vi "Logging Message Loop.vi"(8 "error in (no error)":errorcluster, 10 "Data Queue":refnum<queue>, 11 "Message Queues":T1) -> (0 "error out":errorcluster)   [LabVIEW 2020, in "Logging.lvlib"]
doc: "The message loop subVI to handle messages pertaining to logging data."
uses:
  Logging.lvlib
  MESSAGE_QUEUE/All Message Queues.ctl
  MESSAGE_QUEUE/Message Cluster.ctl
  SETTING/data_Queue.ctl
  Logging Configuration.ctl
  FITS/BigDataFits.ctl
  FITS/ClustBigFilFits.ctl
  FITS/DataTyp_Header.ctl
  MESSAGE_QUEUE/Message Queue.lvlib
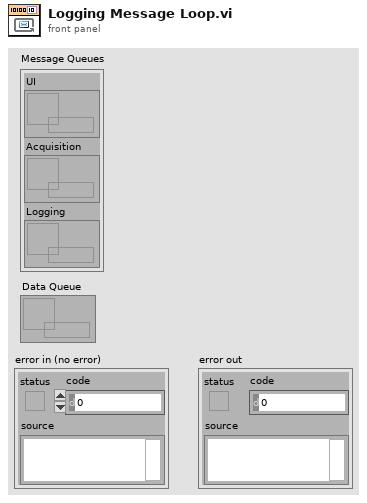
[diagram p1: front panel]
types:
  T1 = typedef "Message Queue.lvlib/All Message Queues.ctl" = cluster{"UI":refnum<queue>, "Acquisition":refnum<queue>, "Logging":refnum<queue>}
  T2 = typedef "Logging.lvlib/Logging Configuration.ctl" = cluster{"Log File Base Path":path, "NbrIma":i32}
  T3 = typedef "DataTyp_Header.ctl" = enum16{"U8 (unsigned integer 8bit)", "I16 (signed integer 16bit)", "U16 (unsigned integer 16 bit)", "I32 (signed integer 32bit)", "U32 (unsigned integer 32 bit)", "SGL (float 32bit)", "DBL(float 64bit)", "complex (2xfloat 64bit)"}
  T4 = typedef "ClustBigFilFits.ctl" = cluster{"file (use dialog)":path, "Type de données":T3, "Commentaire":string, "naxis1":i32, "naxis2":i32, "naxis3":i32, "Exptime":sgl}
  T5 = typedef "BigDataFits.ctl" = enum16{"Init", "WritHeader", "WritData", "Close"}
  T6 = typedef "data_Queue.ctl" = cluster{"tabIma":u16[][], "tabCdG":sgl[], "vectCom":sgl[]}
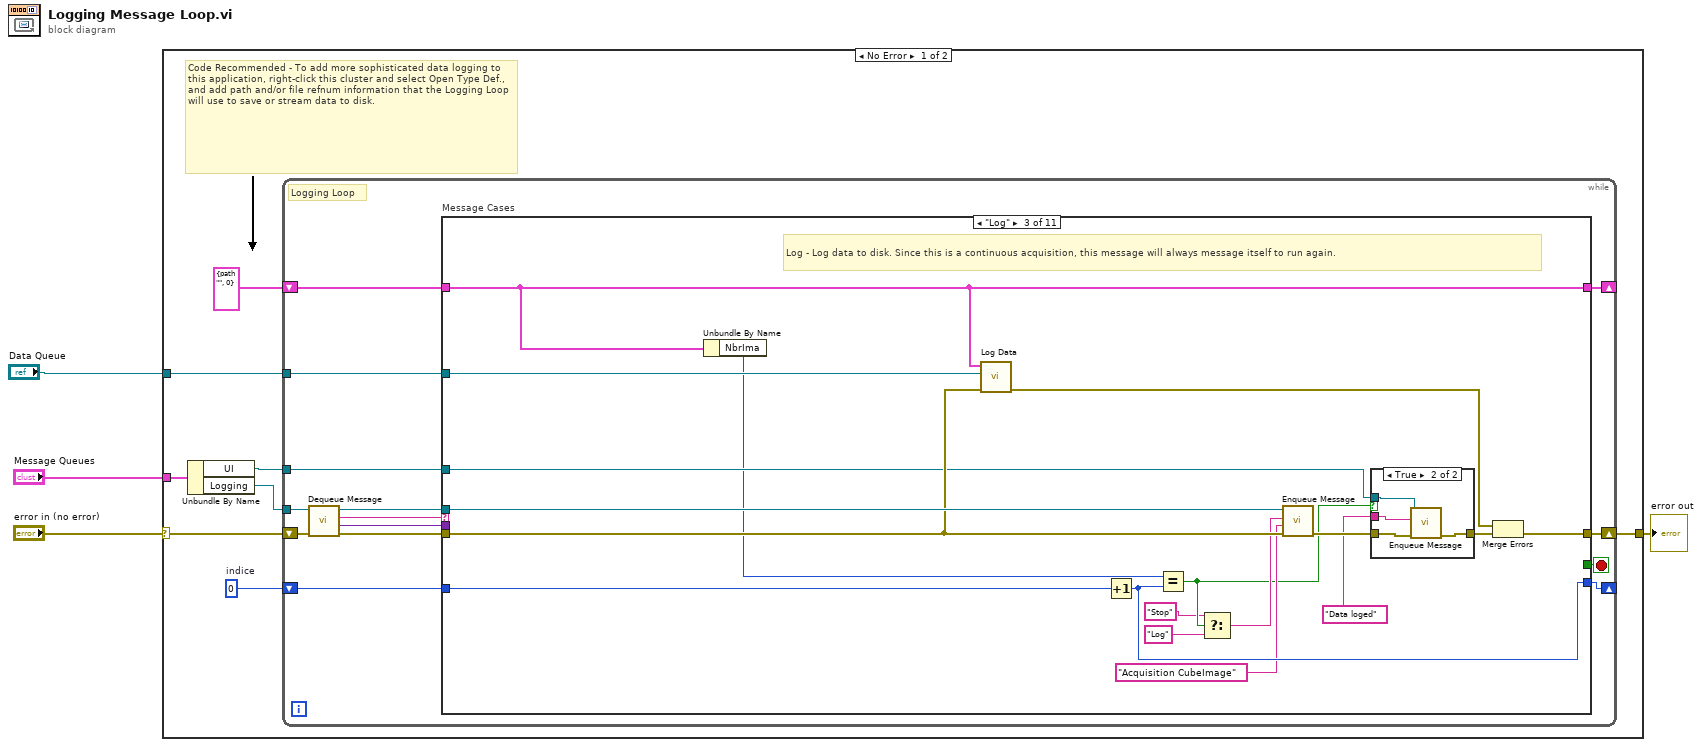
[diagram p0: block diagram]
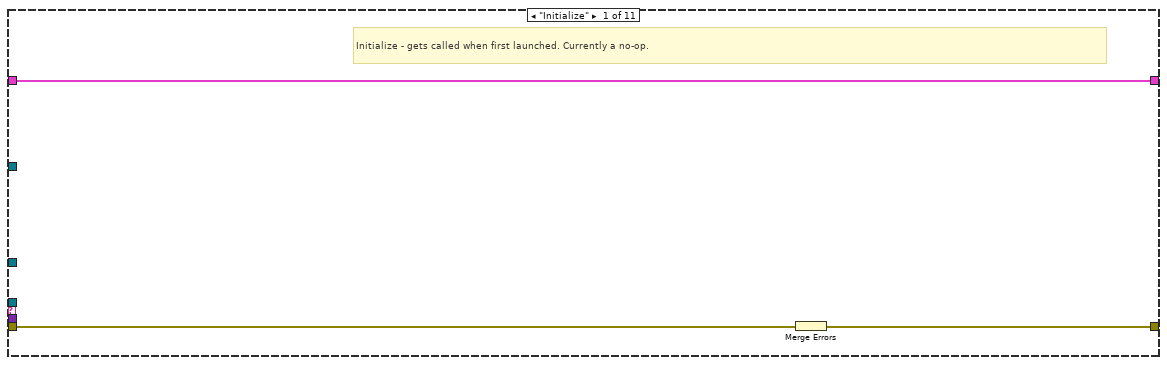
[diagram p2: hidden frame]
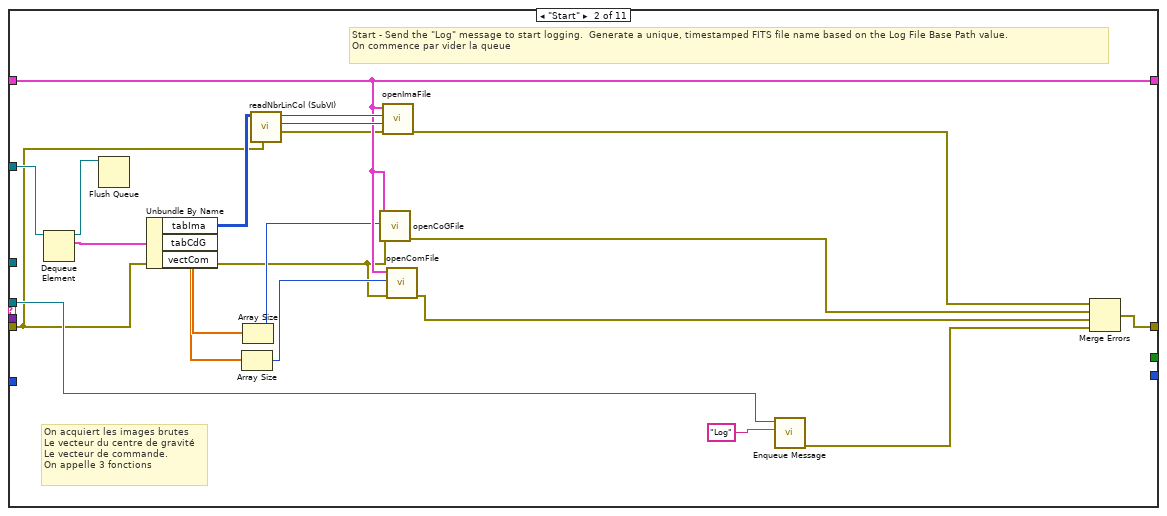
[diagram p3: hidden frame]
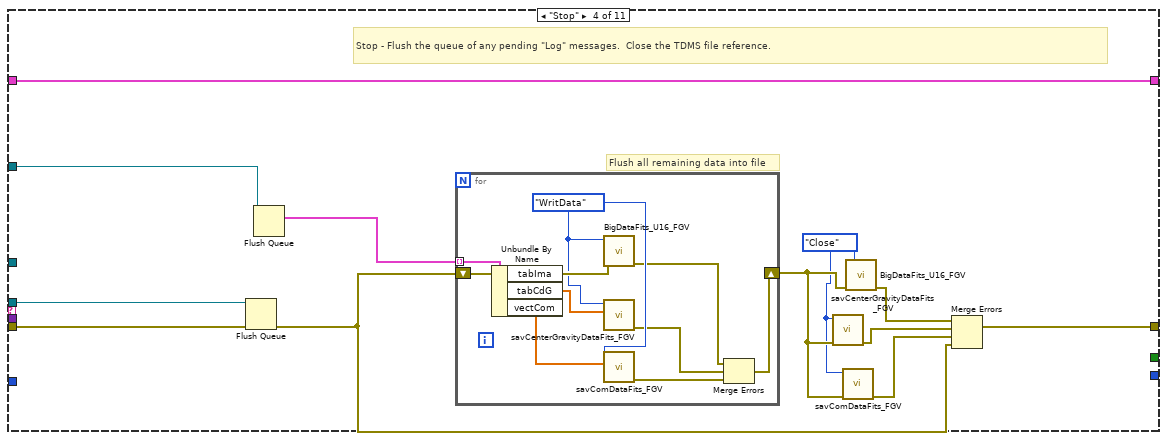
[diagram p5: hidden frame]
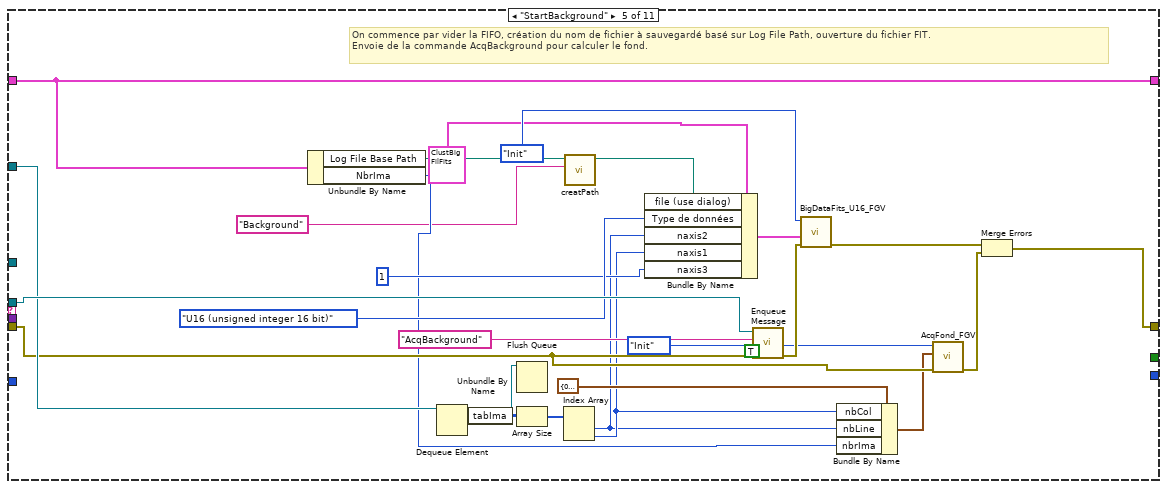
[diagram p6: hidden frame]
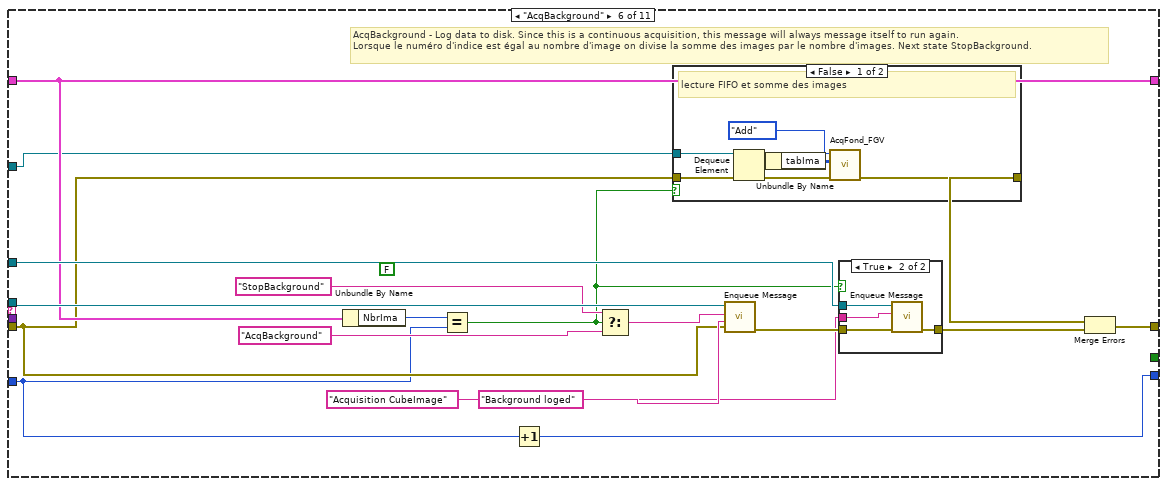
[diagram p7: hidden frame]
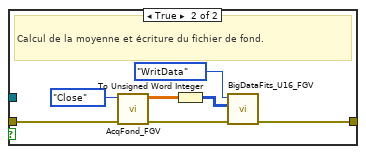
[diagram p8: hidden frame]
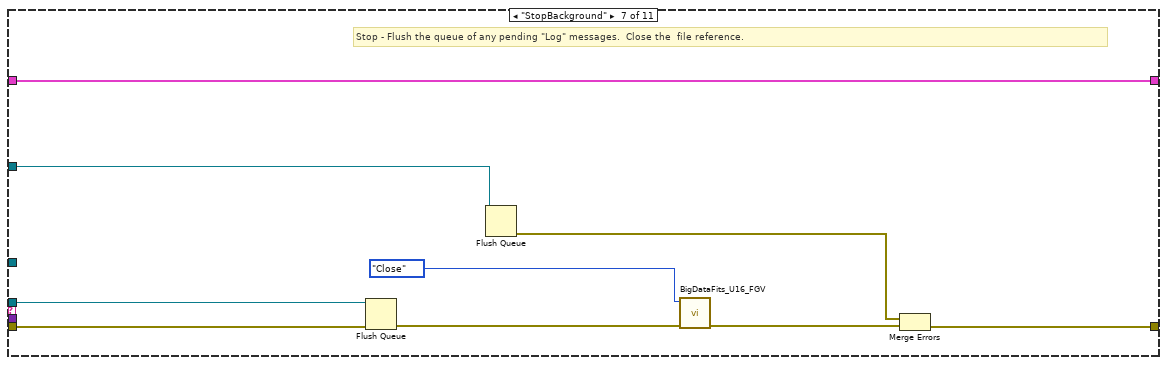
[diagram p10: hidden frame]
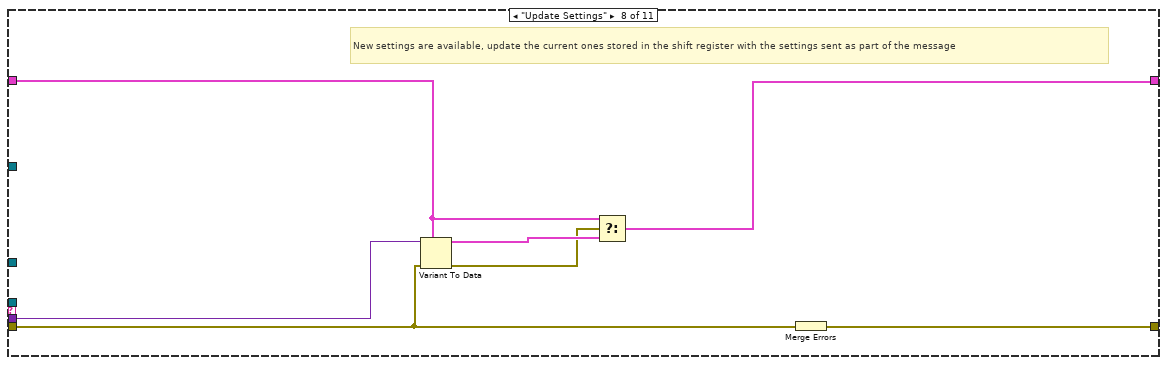
[diagram p11: hidden frame]
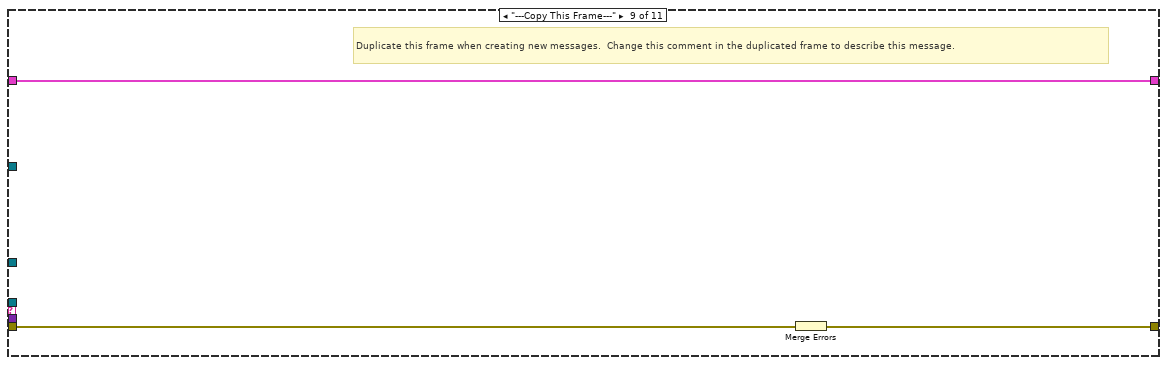
[diagram p12: hidden frame]
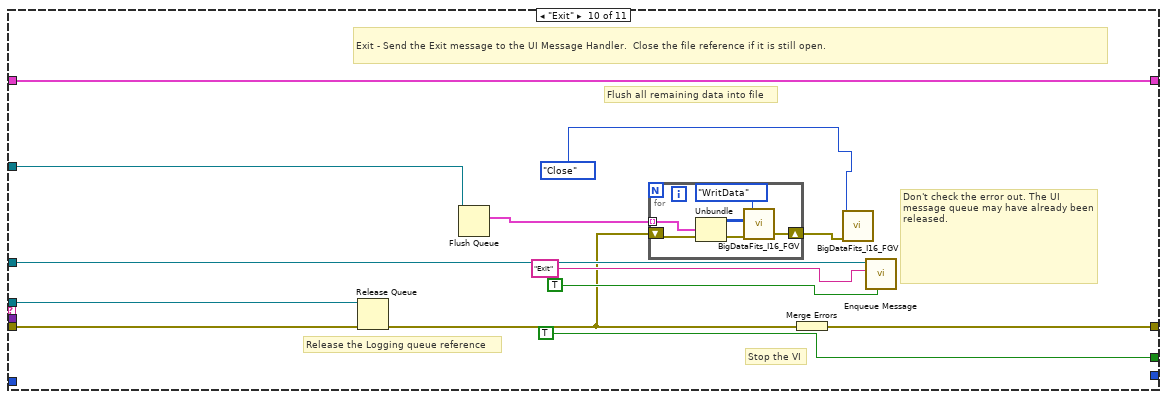
[diagram p13: hidden frame]
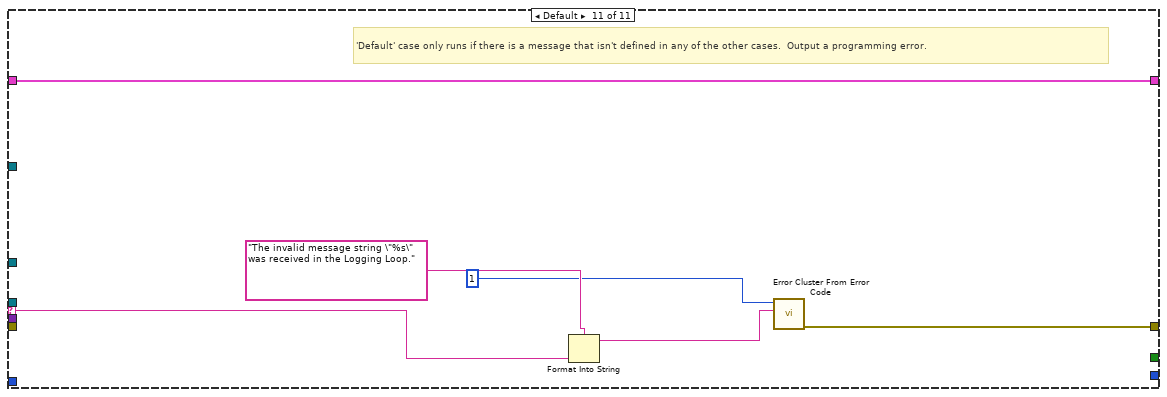
[diagram p14: hidden frame]
diagram:
  n1 = case shown="No Error" "error in (no error)" {
    selector: "error in (no error)" -> [w8 w201]
    tunnel: "Message Queues" -> [w12 _]
    tunnel: [w10 w201] -> w3
    tunnel: "Data Queue" -> [w7 _]
    frame No Error {
      w5 = 0  # indice
      # "Code Recommended - To add more sophisticated data logging to this application, right-click this cluster and select Open Type Def., and add path and/or file refnum information that the Logging Loop will use to save or stream data to disk."
      n2 = Unbundle By Name(w12) -> ("UI"=w6:refnum<queue>, "Logging"=w11:refnum<queue>)
      n3 = while {
        tunnel: w11 -> [w17]
        shift-right: [w25] -> _
        shift-left: T2 {"Log File Base Path"=path "", "NbrIma"=0} ("Logging Configuration") -> [w26]
        shift-right: [w23] -> w10
        shift-left: w8 -> [w22]
        tunnel: w6 -> [w16]
        tunnel: w7 -> [w15]
        shift-right: [w13] -> _
        shift-left: w5 -> [w14]
        stop <- w24 stop-if-true
        # "Logging Loop"
        n4 = call "Dequeue Message.vi"("error in (no error)"=w22, "Message Queue"=w17) -> ("error out"=w21:errorcluster, "Message Data"=w19:variant, "Message"=w20:string, "dup Message Queue"=w18:refnum<queue>)  [unwired: 6 in]
        n5 = case "Message Cases" shown="\"Log\"" w20 {
          selector: w20 -> [_ _ _ _ _ _ _ _ _ _ w198]
          tunnel: w18 -> [_ w47 w65 w81 w119 w137 w164 _ _ w183 _]
          tunnel: w21 -> [w27 w32 w62 w82 w102 w124 w165 w167 w176 w186 _]
          tunnel: [w29 w48 w66 w83 w120 w138 w166 w173 w174 w188 w196] -> w23
          tunnel: w26 -> [w28 w35 w51 w77 w104 w129 w162 w171 w175 w182 w200]
          tunnel: [w28 w35 w51 w77 w104 w129 w162 w168 w175 w182 w200] -> w25
          tunnel: [_ _ _ _ _ _ _ _ _ TRUE _] -> w24
          tunnel: w19 -> [_ _ _ _ _ _ _ w172 _ _ _]
          tunnel: w16 -> [_ _ w54 _ _ w131 _ _ _ w187 _]
          tunnel: w15 -> [_ w42 w64 w80 w109 w125 w163 _ _ w180 _]
          tunnel: w14 -> [_ _ w61 _ _ w122 _ _ _ _ _]
          tunnel: [_ _ w60 _ _ w121 _ _ _ _ _] -> w13
          frame "Initialize" {
            # "Initialize - gets called when first launched. Currently a no-op."
            n6 = Merge Errors(w27) -> (w29:errorcluster)
          }
          frame "Start" {
            # "On acquiert les images brutes \nLe vecteur du centre de gravité\nLe vecteur de commande. \nOn appelle 3 fonctions"
            # "Start - Send the \"Log\" message to start logging.  Generate a unique, timestamped FITS file name based on the Log File Base Path value. \nOn commence par vider la queue"
            n7 = Dequeue Element(queue=w42) -> (queue out=w41:refnum<queue>, element=w40:T6)  [unwired: 2 in, 2 out]
            n8 = Flush Queue(queue=w41) -> ()  [unwired: 1 in, 3 out]
            n9 = Unbundle By Name(w40) -> ("tabIma"=w39:u16[][], "tabCdG"=w38:sgl[], "vectCom"=w37:sgl[])
            n10 = Array Size(array=w37) -> (size(s)=w34:i32)
            n11 = Array Size(array=w38) -> (size(s)=w33:i32)
            n12 = call "readNbrLinCol (SubVI).vi"("tabIma"=w39) -> ("nbrCol"=w43:i32, "nbrLine"=w44:i32)  [unwired: 9 in]
            n13 = call "openCoGFile.vi"("error in (no error)"=w32, "nbrCol"=w33, "Logging Configuration"=w35) -> ("error out"=w31:errorcluster)  [unwired: 8 in]
            n14 = call "openImaFile.vi"("error in (no error)"=w32, "nbrCol"=w43, "nbrLine"=w44, "Logging Configuration"=w35) -> ("error out"=w45:errorcluster)  [unwired: 7 in]
            n15 = call "openComFile.vi"("error in (no error)"=w32, "nbrLine"=w34, "Logging Configuration"=w35) -> ("error out"=w30:errorcluster)  [unwired: 8 in]
            n16 = call "Enqueue Message.vi"("Message"="Log", "Message Queue"=w47) -> ("error out"=w36:errorcluster)  [unwired: 8 in, 1 out]
            n17 = Merge Errors(w45, w31, w30, w36) -> (w48:errorcluster)
          }
          frame "Log" {
            # "Log - Log data to disk. Since this is a continuous acquisition, this message will always message itself to run again."
            n18 = Unbundle By Name(w51) -> ("NbrIma"=w50:i32)
            n19 = call "Log Data.vi"("error in (no error)"=w62, "Data Queue"=w64, "Logging Configuration"=w51) -> ("error out"=w63:errorcluster)  [unwired: 8 in]
            n20 = Increment(x=w61) -> (x+1=w60:i32)
            n21 = Equal?(x=w50, y=w60) -> (x = y?=w53:bool)
            n22 = Select(t="Stop", s=w53, f="Log" ("Message")) -> (s? t:f=w58:string)
            n23 = call "Enqueue Message.vi"("error in (no error)"=w62, "Message Data"="Acquisition CubeImage" ("t"), "Message"=w58, "Message Queue"=w65) -> ("error out"=w56:errorcluster)  [unwired: 6 in, 1 out]
            n24 = case shown="True" w53 {
              tunnel: w56 -> [w67 w71]
              tunnel: [w67 w70] -> w55
              tunnel: w54 -> [_ w69]
              tunnel: "Data loged" ("t") -> [_ w68]
              frame False {
              }
              frame True {
                n25 = call "Enqueue Message.vi"("error in (no error)"=w71, "Message"=w68, "Message Queue"=w69) -> ("error out"=w70:errorcluster)  [unwired: 7 in, 1 out]
              }
            }
            n26 = Merge Errors(w63, w55) -> (w66:errorcluster)
          }
          frame "Stop" {
            w75 = BigDataFits."Close" ("Énum")
            # "Flush all remaining data into file"
            # "Stop - Flush the queue of any pending \"Log\" messages.  Close the TDMS file reference."
            n27 = Flush Queue(queue=w81, error in (no error)=w82) -> (error out=w72:errorcluster)  [unwired: 2 out]
            n28 = Flush Queue(queue=w80) -> (remaining elements=w79:T6[])  [unwired: 1 in, 2 out]
            n29 = for {
              shift-right: [w87] -> w76
              shift-left: w72 -> [w92]
              tunnel: w79 -> [w93] mode=indexing
              w90 = BigDataFits."WritData" ("Énum")
              n30 = Unbundle By Name(w93) -> ("tabIma"=w91:u16[][], "tabCdG"=w89:sgl[], "vectCom"=w88:sgl[])
              n31 = call "BigDataFits_U16_FGV.vi"("InError"=w92, "entier 16 bits"=w91, "Énum"=w90) -> ("sortie d'erreur"=w86:errorcluster)  [unwired: 8 in]
              n32 = call "savCenterGravityDataFits_FGV.vi"("SGL 32 bits"=w89, "Énum"=w90) -> ("sortie d'erreur"=w85:errorcluster)  [unwired: 9 in]
              n33 = call "savComDataFits_FGV.vi"("SGL 32 bits"=w88, "Énum"=w90) -> ("sortie d'erreur"=w84:errorcluster)  [unwired: 9 in]
              n34 = Merge Errors(w86, w85, w84) -> (w87:errorcluster)
            }
            n35 = call "savCenterGravityDataFits_FGV.vi"("InError"=w76, "Énum"=w75) -> ("sortie d'erreur"=w74:errorcluster)  [unwired: 9 in]
            n36 = call "savComDataFits_FGV.vi"("InError"=w76, "Énum"=w75) -> ("sortie d'erreur"=w73:errorcluster)  [unwired: 9 in]
            n37 = call "BigDataFits_U16_FGV.vi"("InError"=w76, "Énum"=w75) -> ("sortie d'erreur"=w78:errorcluster)  [unwired: 9 in]
            n38 = Merge Errors(w78, w74, w73, w72) -> (w83:errorcluster)
          }
          frame "StartBackground" {
            (unwired) TRUE ("Init")
            # "On commence par vider la FIFO, création du nom de fichier à sauvegardé basé sur Log File Path, ouverture du fichier FIT. \nEnvoie de la commande AcqBackground pour calculer le fond."
            n39 = Unbundle By Name(w104) -> ("Log File Base Path"=w117:path, "NbrIma"=w99:i32)
            n40 = Dequeue Element(queue=w109) -> (queue out=w108:refnum<queue>, element=w105:T6)  [unwired: 2 in, 2 out]
            n41 = Unbundle By Name(w105) -> ("tabIma"=w94:u16[][])
            n42 = Flush Queue(queue=w108) -> ()  [unwired: 1 in, 3 out]
            n43 = Array Size(array=w94) -> (size(s)=w110:i32[])
            n44 = Index Array(array=w110) -> (element #1=w96:i32, element #2=w97:i32)  [unwired: 2 in]
            n45 = call "creatPath.vi"("string"="Background", "Log File Base Path"=w117) -> ("appended path"=w111:path)  [unwired: 9 in]
            n46 = Bundle By Name(cluster=T4 {"file (use dialog)"=path "D:/DATA/Imatest.fits", "Type de données"=enum."U16 (unsigned integer 16 bit)", "Commentaire"="", "naxis1"=0, "naxis2"=0, "naxis3"=1, "Exptime"=1.0} ("ClustBigFilFits"), "file (use dialog)"=w111, "Type de données"=DataTyp_Header."U16 (unsigned integer 16 bit)", "naxis2"=w96, "naxis1"=w97, "naxis3"=1) -> (w113:T4)
            n47 = call "Enqueue Message.vi"("error in (no error)"=w102, "Message"="AcqBackground", "Message Queue"=w119) -> ("error out"=w115:errorcluster)  [unwired: 7 in, 1 out]
            n48 = call "BigDataFits_U16_FGV.vi"("InError"=w115, "ClustBigFilFits"=w113, "Énum"=BigDataFits."Init") -> ("sortie d'erreur"=w116:errorcluster)  [unwired: 8 in]
            n49 = Bundle By Name(cluster=cluster{"nbLine":i32, "nbCol":i32, "nbrIma":i32} {"nbLine"=0, "nbCol"=0, "nbrIma"=0} ("Cluster"), "nbCol"=w97, "nbLine"=w96, "nbrIma"=w99) -> (w98:cluster{"nbLine":i32, "nbCol":i32, "nbrIma":i32})
            n50 = call "AcqFond_FGV.vi"("Error In"=w102, "Cluster"=w98, "Enum"=enum16{"Init", "Add", "Close"}."Init") -> ("Error Out"=w101:errorcluster)  [unwired: 7 in, 1 out]
            n51 = Merge Errors(w116, w101) -> (w120:errorcluster)
          }
          frame "AcqBackground" {
            (unwired) FALSE ("x = y?")
            # "AcqBackground - Log data to disk. Since this is a continuous acquisition, this message will always message itself to run again.\nLorsque le numéro d'indice est égal au nombre d'image on divise la somme des images par le nombre d'images. Next state StopBackground."
            n52 = Unbundle By Name(w129) -> ("NbrIma"=w126:i32)
            n53 = Equal?(x=w126, y=w122) -> (x = y?=w127:bool)
            n54 = Increment(x=w122) -> (x+1=w121:i32)
            n55 = Select(t="StopBackground", s=w127, f="AcqBackground" ("Message")) -> (s? t:f=w135:string)
            n56 = case shown="False" w127 {
              tunnel: w125 -> [w142 _]
              tunnel: w124 -> [w141 w147]
              tunnel: [w140 w146] -> w123
              frame False {
                # "lecture FIFO et somme des images"
                n57 = Dequeue Element(queue=w142, error in (no error)=w141) -> (element=w143:T6, error out=w144:errorcluster)  [unwired: 1 in, 2 out]
                n58 = Unbundle By Name(w143) -> ("tabIma"=w139:u16[][])
                n59 = call "AcqFond_FGV.vi"("Error In"=w144, "Image"=w139, "Enum"=enum16{"Init", "Add", "Close"}."Add") -> ("Error Out"=w140:errorcluster)  [unwired: 7 in, 1 out]
              }
              frame True {
                # "Calcul de la moyenne et écriture du fichier de fond."
                n60 = call "AcqFond_FGV.vi"("Error In"=w147, "Enum"=enum16{"Init", "Add", "Close"}."Close") -> ("Error Out"=w149:errorcluster, "fond"=w150:dbl[][])  [unwired: 8 in]
                n61 = To Unsigned Word Integer(number=w150) -> (unsigned 16bit integer=w148:u16[][])
                n62 = call "BigDataFits_U16_FGV.vi"("InError"=w149, "entier 16 bits"=w148, "Énum"=BigDataFits."WritData") -> ("sortie d'erreur"=w146:errorcluster)  [unwired: 8 in]
              }
            }
            n63 = call "Enqueue Message.vi"("error in (no error)"=w124, "Message Data"="Acquisition CubeImage" ("t"), "Message"=w135, "Message Queue"=w137) -> ("error out"=w133:errorcluster)  [unwired: 6 in, 1 out]
            n64 = case shown="True" w127 {
              tunnel: w133 -> [w153 w157]
              tunnel: [w153 w156] -> w132
              tunnel: w131 -> [_ w155]
              tunnel: "Background loged" ("t") -> [_ w154]
              frame False {
              }
              frame True {
                n65 = call "Enqueue Message.vi"("error in (no error)"=w157, "Message"=w154, "Message Queue"=w155) -> ("error out"=w156:errorcluster)  [unwired: 7 in, 1 out]
              }
            }
            n66 = Merge Errors(w123, w132) -> (w138:errorcluster)
          }
          frame "StopBackground" {
            # "Stop - Flush the queue of any pending \"Log\" messages.  Close the  file reference."
            n67 = Flush Queue(queue=w164, error in (no error)=w165) -> (error out=w159:errorcluster)  [unwired: 2 out]
            n68 = Flush Queue(queue=w163) -> (error out=w161:errorcluster)  [unwired: 1 in, 2 out]
            n69 = call "BigDataFits_U16_FGV.vi"("InError"=w159, "Énum"=BigDataFits."Close") -> ("sortie d'erreur"=w158:errorcluster)  [unwired: 9 in]
            n70 = Merge Errors(w161, w158) -> (w166:errorcluster)
          }
          frame "Update Settings" {
            # "New settings are available, update the current ones stored in the shift register with the settings sent as part of the message"
            n71 = Variant To Data(error in=w167, type=w171, Variant=w172) -> (data=w170:T2, error out=w169:errorcluster)
            n72 = Select(t=w171, s=w169, f=w170) -> (s? t:f=w168:T2)
            n73 = Merge Errors(w167) -> (w173:errorcluster)
          }
          frame "---Copy This Frame---" {
            # "Duplicate this frame when creating new messages.  Change this comment in the duplicated frame to describe this message."
            n74 = Merge Errors(w176) -> (w174:errorcluster)
          }
          frame "Exit" {
            # "Flush all remaining data into file"
            # "Release the Logging queue reference"
            # "Don't check the error out. The UI message queue may have already been released."
            # "Stop the VI"
            # "Exit - Send the Exit message to the UI Message Handler.  Close the file reference if it is still open."
            n75 = Release Queue(queue=w183, error in (no error)=w186) -> (error out=w179:errorcluster)  [unwired: 1 in, 2 out]
            n76 = Flush Queue(queue=w180) -> (remaining elements=w181:T6[])  [unwired: 1 in, 2 out]
            n77 = for {
              shift-right: [w191] -> w177
              shift-left: w179 -> [w190]
              tunnel: w181 -> [w194] mode=indexing
              n78 = Unbundle(w194) -> ("tabIma"=w192:u16[][])  [unwired: 2 out]
              n79 = call "BigDataFits_I16_FGV.vi"("InError"=w190, "entier 16 bits"=w192, "Énum"=BigDataFits."WritData") -> ("sortie d'erreur"=w191:errorcluster)  [unwired: 8 in]
            }
            n80 = Merge Errors(w179) -> (w188:errorcluster)
            n81 = call "BigDataFits_I16_FGV.vi"("InError"=w177, "Énum"=BigDataFits."Close") -> ()  [unwired: 9 in, 1 out]
            n82 = call "Enqueue Message.vi"("Priority Message? (F)"=TRUE, "Message"="Exit", "Message Queue"=w187) -> ()  [unwired: 7 in, 2 out]
          }
          frame Default {
            # "'Default' case only runs if there is a message that isn't defined in any of the other cases.  Output a programming error."
            n83 = Format Into String(format string="The invalid message string \"%s\" was received in the Logging Loop." ("Invalid Logging Message"), w198) -> (resulting string=w195:string)  [unwired: 2 in, 1 out]
            n84 = call <vilib>:"Error Cluster From Error Code.vi"("error message (\"\")"=w195, "error code (0)"=1) -> ("error out"=w196:errorcluster)  [unwired: 7 in]
          }
        }
      }
    }
    frame Error {
    }
  }
  "error out" <- w3
